vi "DoubleCoincidencesCheck_sort_data.vi"(10 "initialized array":dbl[][](array[numeric]), 11 "Cluster In in":T1 {"Coincidence Window" format="%#_13g"; "Delay12" format="%#_13g"; "Delay02" format="%#_13g"; "Delay01" format="%#_13g"}) -> (3 "Cluster In out":T1 {"Coincidence Window" format="%#_13g"; "Delay12" format="%#_13g"; "Delay02" format="%#_13g"; "Delay01" format="%#_13g"})   [LabVIEW 2023]
uses:
  Get_Delays_Ctrl.ctl
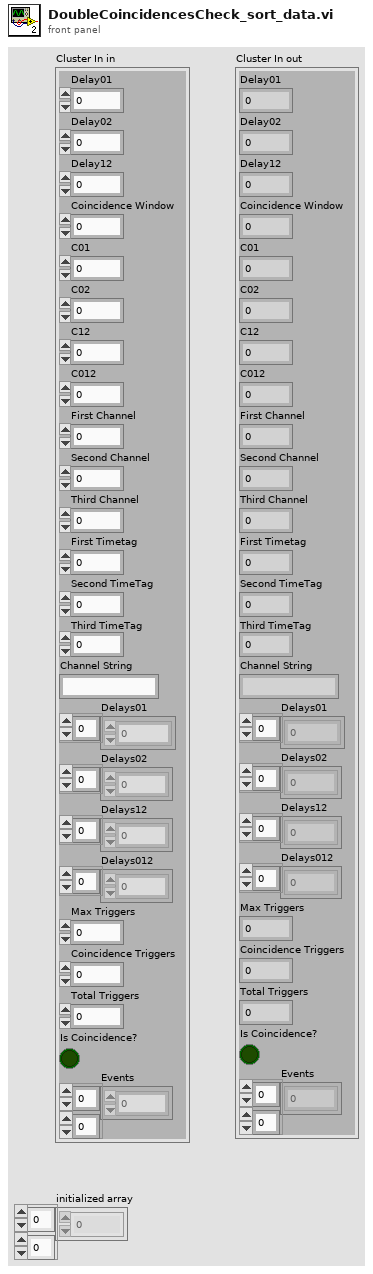
[diagram p1: front panel]
types:
  T1 = typedef "Get_Delays_Ctrl.ctl" = cluster{"Delay01":dbl, "Delay02":dbl, "Delay12":dbl, "Coincidence Window":dbl, "C01":u32, "C02":u32, "C12":u32, "C012":u32, "First Channel":dbl, "Second Channel":dbl, "Third Channel":dbl, "First Timetag":dbl, "Second TimeTag":dbl, "Third TimeTag":dbl, "Channel String":string, "Delays01":sgl[], "Delays02":dbl[], "Delays12":dbl[], "Delays012":dbl[], "Max Triggers":i32, "Coincidence Triggers":i32, "Total Triggers":i32, "Is Coincidence?":bool, "Events":u64[][]}
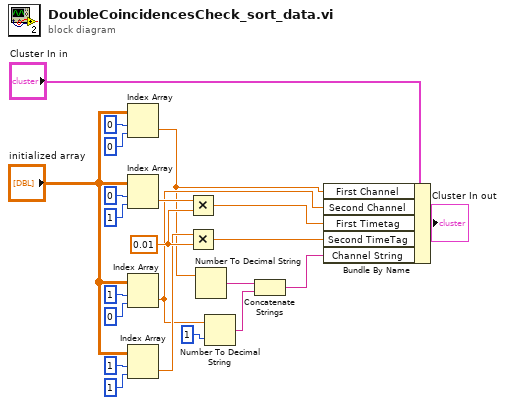
[diagram p0: block diagram]
diagram:
  w21 = 0.01 ("y")
  n1 = Index Array(array="initialized array", index (row)=0, index (col)=0 ("disabled index (col)")) -> (element=w14:dbl)
  n2 = Index Array(array="initialized array", index (row)=0, index (col)=1 ("disabled index (col)")) -> (element=w18:dbl)
  n3 = Index Array(array="initialized array", index (row)=1, index (col)=0 ("disabled index (col)")) -> (element=w16:dbl)
  n4 = Index Array(array="initialized array", index (row)=1, index (col)=1 ("disabled index (col)")) -> (element=w20:dbl)
  n5 = Multiply(x=w18, y=w21) -> (x*y=w19:dbl)
  n6 = Multiply(x=w20, y=w21) -> (x*y=w22:dbl)
  n7 = Number To Decimal String(number=w14) -> (decimal integer string=w12:string)  [unwired: 1 in]
  n8 = Number To Decimal String(number=w16, width (-)=i16 1) -> (decimal integer string=w11:string)
  n9 = Concatenate Strings(w12, w11) -> (w15:string)
  n10 = Bundle By Name(cluster="Cluster In in", "First Channel"=w14, "Second Channel"=w16, "First Timetag"=w19, "Second TimeTag"=w22, "Channel String"=w15) -> (→"Cluster In out":T1)
